vi "GenFade.vi"(5 "End Color":u32(colorbox), 6 "Reset":bool, 7 "Start Color":u32(colorbox), 10 "Total Time (ms)":u32, 11 "NumLeds":i32) -> (2 "Finished":bool, 3 "Array":u32[](array[numeric]))   [LabVIEW 2020, in "ArduinoSerialBling.lvlib"]
uses:
  ArduinoSerialBling.lvlib
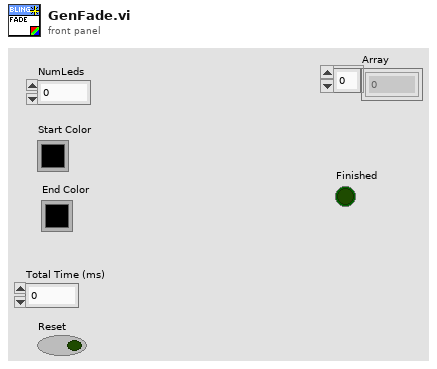
[diagram p1: front panel]
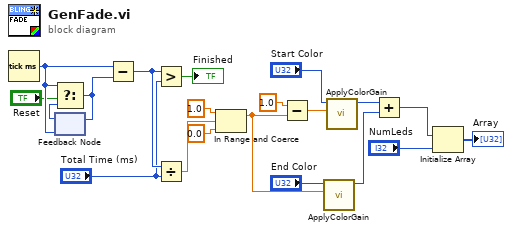
[diagram p0: block diagram]
diagram:
  n1 = Tick Count (ms)() -> (millisecond timer value=w18:u32)
  n2 = feedback #1(w18) -> (w20:u32)
  n3 = Select(t=w18, s="Reset", f=w20) -> (s? t:f=w19:u32)
  n4 = feedback-in #1(w19) -> ()
  n5 = Subtract(x=w18, y=w19) -> (x-y=w17:u32)
  n6 = Greater?(x=w17, y="Total Time (ms)") -> (0:→"Finished":bool)
  n7 = Divide(x=w17, y="Total Time (ms)") -> (x/y=w12:dbl)
  n8 = In Range and Coerce(upper limit=1.0, x=w12, lower limit=0.0) -> (coerced(x)=w9:dbl)  [unwired: 1 out]
  n9 = Subtract(x=1.0, y=w9) -> (x-y=w10:dbl)
  n10 = call "ApplyColorGain.vi"("Gain"=w9, "Color In"="End Color") -> ("Color Out"=w5:u32)  [unwired: 9 in]
  n11 = call "ApplyColorGain.vi"("Gain"=w10, "Color In"="Start Color") -> ("Color Out"=w6:u32)  [unwired: 9 in]
  n12 = Add(x=w6, y=w5) -> (x+y=w4:u32)
  n13 = Initialize Array(w4, "NumLeds") -> (→"Array":u32[])
